vi "Configure Totalizer.vi"(0 "VISA resource name":refnum<visa-resource-name>, 5 "Totalizer Channel (125)":string="125", 7 "Reset After Read (False)":bool, 9 "Signal Edge (0: Rising)":u16(ring) items=["Rising", "Falling"], 11 "error in (no error)":errorcluster) -> (4 "VISA resource name out":refnum<visa-resource-name>, 15 "error out":errorcluster)   [LabVIEW 2020, in "Keithley 27XX.lvlib"]
doc: "This VI allows you to control the reset behavior of the totalizer channel of a plug in module. It also provides configuration for the type of edge to count."
uses:
  <instrlib>/Keithley 27XX/Keithley 27XX.lvlib
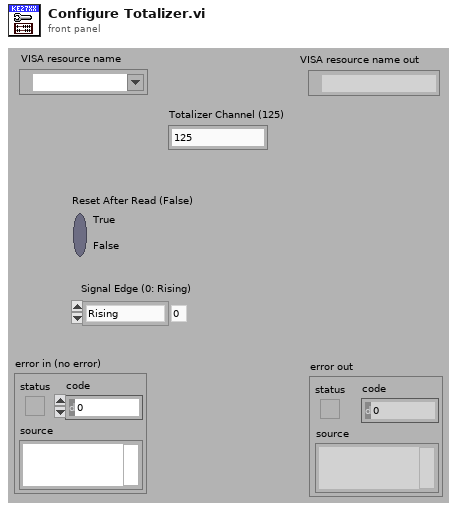
[diagram p1: front panel]
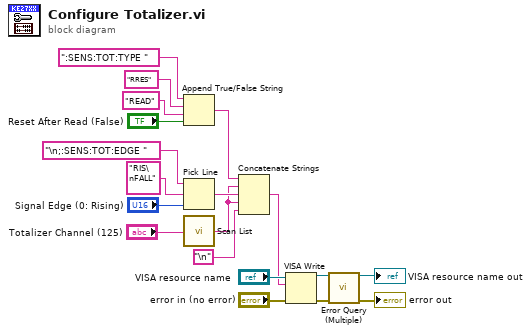
[diagram p0: block diagram]
diagram:
  n1 = Append True/False String(1:"Reset After Read (False)", 2:"READ" ("true string"), 3:"RRES" ("false string"), 4:":SENS:TOT:TYPE " ("string (\"\")")) -> (0:w13:string)
  n2 = Pick Line(string ("")="\n;:SENS:TOT:EDGE ", multi-line string="RIS\nFALL" ("true string"), line index="Signal Edge (0: Rising)") -> (output string=w12:string)
  n3 = call <instrlib>:"Scan List.vi"("Scan List (Empty)"="Totalizer Channel (125)") -> ("Scan List Out"=w11:string)  [unwired: 14 in]
  n4 = Concatenate Strings(w13, w11, w12, w11, "\n") -> (w10:string)
  n5 = VISA Write(VISA resource name="VISA resource name", write buffer=w10, error in (no error)="error in (no error)") -> (VISA resource name out=w9:refnum<visa-resource-name>, error out=w8:errorcluster)  [unwired: 1 out]
  n6 = call <instrlib>:"Error Query (Multiple).vi"("VISA resource name"=w9, "error in (no error)"=w8) -> ("VISA resource name out"=→"VISA resource name out":refnum<visa-resource-name>, "error out"=→"error out":errorcluster)  [unwired: 10 in, 2 out]
